vi "Ionizer_Monitor_test.vi"() -> ()   [LabVIEW 2016]
panel:
  in  "Tab Control":T1(tab)
  out "Oven Temperature 2":dbl(graph)
  out "Magnet Field":dbl(graph)
  out "field value:":dbl
  out "Oven Temp:":dbl
  out "Omega read buffer":string
  out "Group3 read buffer":string
  in  "stop":bool
  in  "Group 3 VISA resource":refnum<visa-resource-name>="TCPIP0::192.168.1.160::966::SOCKET"
  in  "byte count 2":u32=15
  in  "Loop multiple (ms)":u32=500
  in  "Wait (ms)":u32=500
  in  "byte count":u32=15
  in  "Omega VISA resource":refnum<visa-resource-name>="TCPIP0::192.168.1.160::966::SOCKET"
  out "Omega T error":errorcluster
  out "Group3 Error":errorcluster
  out "Read errors":i32
  out "Group3 Iteration":i32
  out "Omega Iteration":i32
  # "°C"
  # "T"
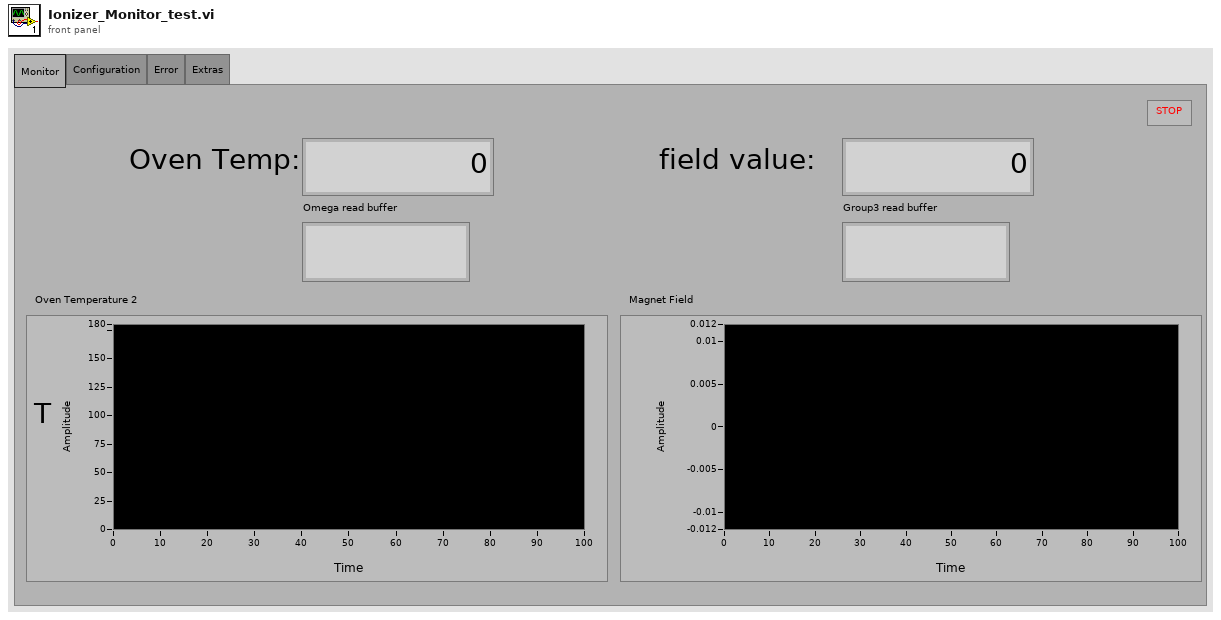
[diagram p1: front panel]
types:
  T1 = enum32{"Monitor", "Configuration", "Error", "Extras"}
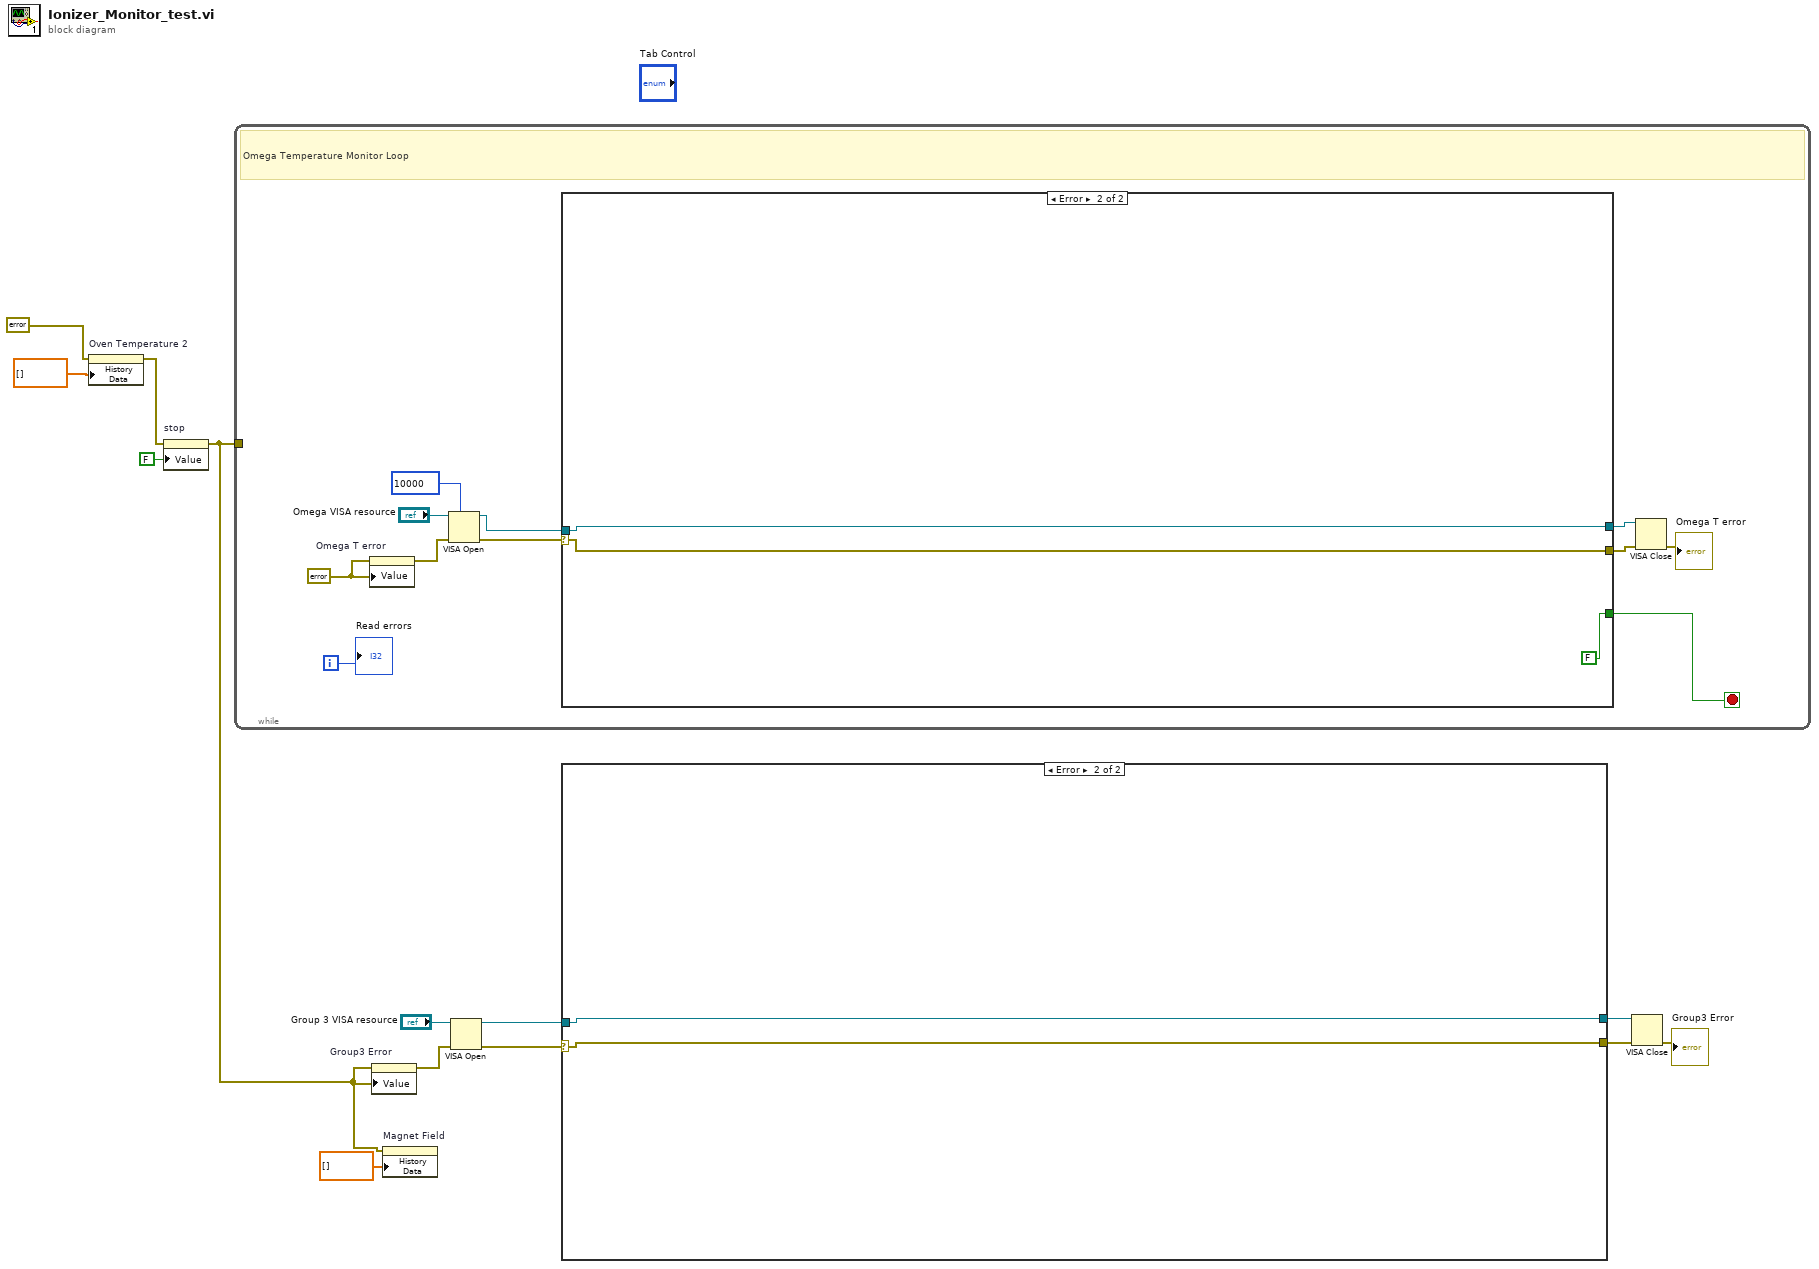
[diagram p0: block diagram]
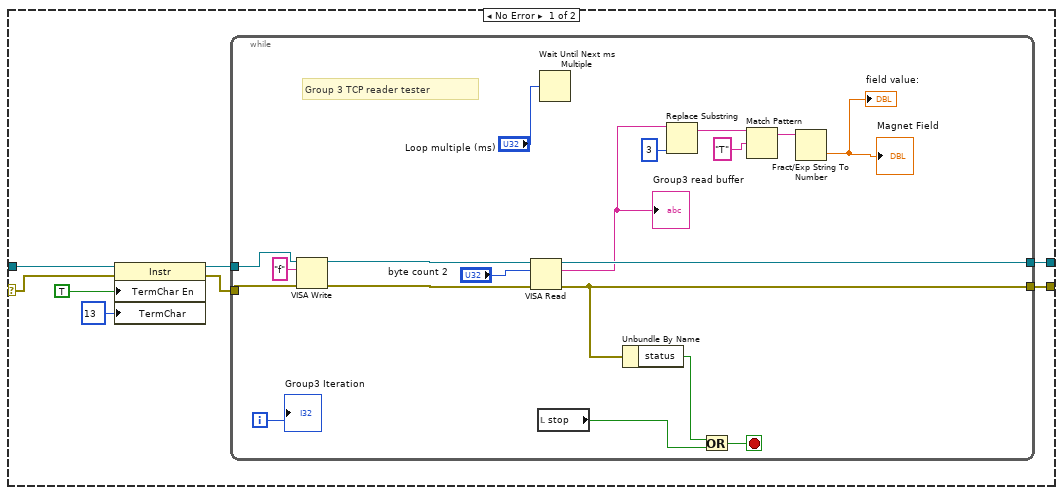
[diagram p2: hidden frame]
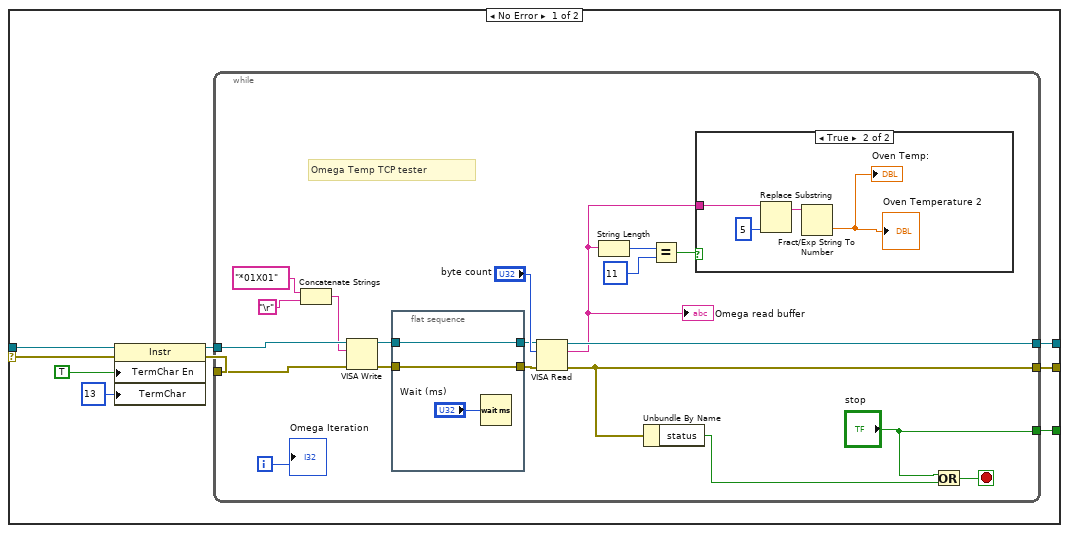
[diagram p3: hidden frame]
diagram:
  n1 = property on="Oven Temperature 2" class="WFChart (strict)"(error in=errorcluster {"status"=FALSE, "code"=0, "source"=""} ("error in (no error)"), "History Data"=dbl[] []) -> (error out=w3:errorcluster)  [unwired: 1 in, 1 out]
  n2 = property on="stop" class="Bool (strict)"(error in=w3, "Value"=FALSE ("stop")) -> (error out=w1:errorcluster)  [unwired: 1 in, 1 out]
  n3 = while {
    tunnel: w1 -> [_]
    i -> [w14]
    stop <- w15 stop-if-true
    w17 = errorcluster {"status"=FALSE, "code"=0, "source"=""} ("error in (no error)")
    # "Omega Temperature Monitor Loop"
    n4 = property on="Omega T error" class="Clust (strict)"(error in=w17, "Value"=w17) -> (error out=w19:errorcluster)  [unwired: 1 in, 1 out]
    n5 = VISA Open(timeout (0)=u32 10000 ("VISA Open timeout (0)"), error in (no error)=w19, VISA resource name="Omega VISA resource") -> (VISA resource name=w24:refnum<visa-resource-name>, error out=w20:errorcluster)  [unwired: 2 in]
    n6 = case shown="Error" w20 {
      selector: w20 -> [w25 w61]
      tunnel: w24 -> [w31 w63]
      tunnel: [w33 w63] -> w23
      tunnel: [w32 w61] -> w22
      tunnel: [w26 FALSE ("stop")] -> w15
      frame No Error {
        n7 = property class="Instr"(reference=w31, error in=w25, "TermChar En"=TRUE ("Message Based Settings:Termination Character Enable"), "TermChar"=u8 13 ("Message Based Settings:Termination Character")) -> (reference out=w30:refnum<visa-resource-name>, error out=w29:errorcluster)
        n8 = while {
          tunnel: w30 -> [w49]
          tunnel: [w53] -> w33
          tunnel: w29 -> [w44]
          tunnel: [w52] -> w32
          tunnel: ["stop"] -> w26
          i -> [w50]
          stop <- w51 stop-if-true
          # "Omega Temp TCP tester"
          n9 = Concatenate Strings("*01X01" ("data in"), "\r") -> (w46:string)
          n10 = VISA Write(VISA resource name=w49, write buffer=w46, error in (no error)=w44) -> (VISA resource name out=w37:refnum<visa-resource-name>, error out=w39:errorcluster)  [unwired: 1 out]
          n11 = flat-sequence {
            tunnel: w39 -> [w56]
            tunnel: [w56] -> w38
            tunnel: w37 -> [w55]
            tunnel: [w55] -> w36
            frame #0 {
              n12 = Wait (ms)(milliseconds to wait="Wait (ms)") -> ()  [unwired: 1 out]
            }
          }
          n13 = VISA Read(VISA resource name=w36, byte count="byte count", error in (no error)=w38) -> (VISA resource name out=w53:refnum<visa-resource-name>, read buffer=w40:string, error out=w52:errorcluster)  [unwired: 1 out]
          "Omega read buffer" <- w40
          n14 = String Length(string=w40) -> (length=w43:i32)
          n15 = Unbundle By Name(w52) -> ("status"=w35:bool)
          n16 = Equal?(x=w43, y=11) -> (x = y?=w41:bool)
          n17 = case shown="True" w41 {
            tunnel: w40 -> [_ w57]
            frame False {
            }
            frame True {
              n18 = Replace Substring(2:5 ("length (len. of substring)"), 5:w57) -> (1:w58:string)  [unwired: 2 in, 1 out]
              n19 = Fract/Exp String To Number(string=w58) -> (number=→"Oven Temp:" →"Oven Temperature 2":dbl)  [unwired: 3 in, 1 out]
            }
          }
          n20 = Or(x="stop", y=w35) -> (x .or. y?=w51:bool)
          "Omega Iteration" <- w50
        }
      }
      frame Error {
      }
    }
    n21 = VISA Close(VISA resource name=w23, error in (no error)=w22) -> (error out=→"Omega T error":errorcluster)
    "Read errors" <- w14
  }
  n22 = property on="Group3 Error" class="Clust (strict)"(error in=w1, "Value"=w1) -> (error out=w7:errorcluster)  [unwired: 1 in, 1 out]
  n23 = property on="Magnet Field" class="WFChart (strict)"(error in=w1, "History Data"=dbl[] []) -> ()  [unwired: 1 in, 2 out]
  n24 = VISA Open(error in (no error)=w7, VISA resource name="Group 3 VISA resource") -> (VISA resource name=w12:refnum<visa-resource-name>, error out=w8:errorcluster)  [unwired: 3 in]
  n25 = case shown="Error" w8 {
    selector: w8 -> [w64 w91]
    tunnel: w12 -> [w69 w92]
    tunnel: [w71 w92] -> w11
    tunnel: [w70 w91] -> w10
    frame No Error {
      n26 = property class="Instr"(reference=w69, error in=w64, "TermChar En"=TRUE ("Message Based Settings:Termination Character Enable"), "TermChar"=u8 13 ("Message Based Settings:Termination Character")) -> (reference out=w68:refnum<visa-resource-name>, error out=w67:errorcluster)
      n27 = while {
        tunnel: w68 -> [w80]
        tunnel: [w88] -> w71
        tunnel: w67 -> [w87]
        tunnel: [w84] -> w70
        i -> [w81]
        stop <- w82 stop-if-true
        # "Group 3 TCP reader tester"
        n28 = VISA Write(VISA resource name=w80, write buffer="f" ("data in"), error in (no error)=w87) -> (VISA resource name out=w89:refnum<visa-resource-name>, error out=w86:errorcluster)  [unwired: 1 out]
        n29 = VISA Read(VISA resource name=w89, byte count="byte count 2", error in (no error)=w86) -> (VISA resource name out=w88:refnum<visa-resource-name>, read buffer=w74:string, error out=w84:errorcluster)  [unwired: 1 out]
        "Group3 read buffer" <- w74
        n30 = local read "stop"() -> (w72:bool)
        n31 = Wait Until Next ms Multiple(millisecond multiple="Loop multiple (ms)") -> ()  [unwired: 1 out]
        n32 = Unbundle By Name(w84) -> ("status"=w83:bool)
        n33 = Replace Substring(2:3 ("length (len. of substring)"), 5:w74) -> (1:w76:string)  [unwired: 2 in, 1 out]
        n34 = Or(x=w83, y=w72) -> (x .or. y?=w82:bool)
        n35 = Match Pattern(string=w76, regular expression="T") -> (before substring=w77:string)  [unwired: 1 in, 3 out]
        n36 = Fract/Exp String To Number(string=w77) -> (number=→"field value:" →"Magnet Field":dbl)  [unwired: 3 in, 1 out]
        "Group3 Iteration" <- w81
      }
    }
    frame Error {
    }
  }
  n37 = VISA Close(VISA resource name=w11, error in (no error)=w10) -> (error out=→"Group3 Error":errorcluster)
